vi "Configure Analog Output.vi"(6 "Enable Analog Output Reference (F: Disable)":bool, 7 "Analog Output Offset (0)":dbl, 8 "error in (no error)":errorcluster, 9 "Analog Output Gain (1)":dbl=1.0, 10 "Enable Analog Output (T: Enable)":bool=TRUE, 11 "VISA resource name":refnum<visa-resource-name>) -> (0 "error out":errorcluster, 3 "VISA resource name out":refnum<visa-resource-name>)   [LabVIEW 2011, in "Keithley 2182.lvlib"]
doc: "Configures the instrument's analog output. The analog output provides a scaled, non-inverting voltage output up to -1.2V and +1.2V. It is typically used to drive a chart recorder.\n\nThe Analog Output voltage is calculated as follows:\n\n<B>Analog Output = (Gain x Rdg/Rng) - Offset</B>\n\nwhere:\n<B>Gain</B> is the user entered gain factor.\n<B>Rdg</B> is the reading on the Model 2182.\n<B>Rng</B> is the measurement range.\n<B>Offset</B> is the user entered offset value."
uses:
  Keithley 2182.lvlib
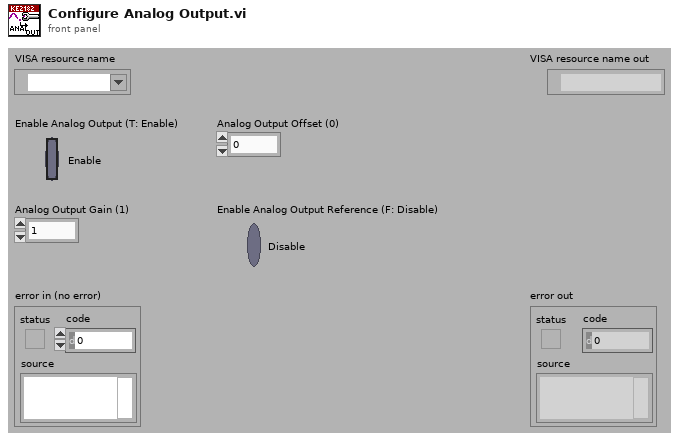
[diagram p1: front panel]
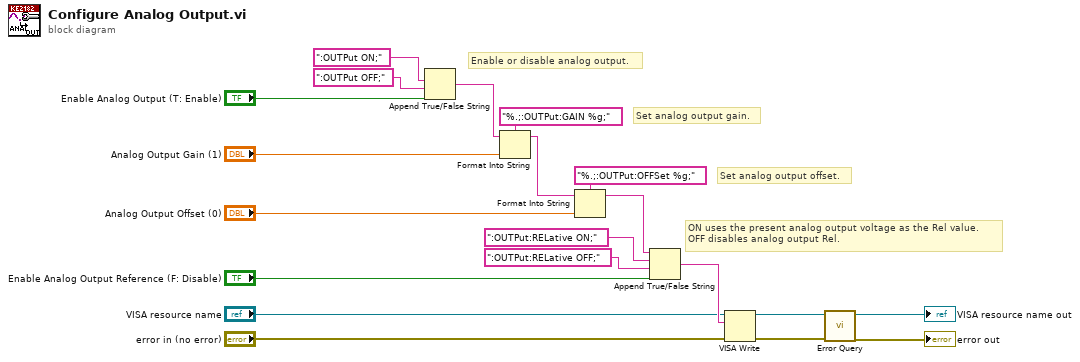
[diagram p0: block diagram]
diagram:
  # "ON uses the present analog output voltage as the Rel value.\nOFF disables analog output Rel."
  # "Set analog output offset."
  # "Set analog output gain."
  # "Enable or disable analog output."
  n1 = Append True/False String(1:"Enable Analog Output (T: Enable)", 2:":OUTPut OFF;", 3:":OUTPut ON;") -> (0:w17:string)  [unwired: 1 in]
  n2 = Format Into String(format string="%.;:OUTPut:GAIN %g;", initial string=w17, "Analog Output Gain (1)") -> (resulting string=w14:string)  [unwired: 1 in, 1 out]
  n3 = Format Into String(format string="%.;:OUTPut:OFFSet %g;", initial string=w14, "Analog Output Offset (0)") -> (resulting string=w11:string)  [unwired: 1 in, 1 out]
  n4 = Append True/False String(1:"Enable Analog Output Reference (F: Disable)", 2:":OUTPut:RELative OFF;", 3:":OUTPut:RELative ON;", 4:w11) -> (0:w7:string)
  n5 = VISA Write(VISA resource name="VISA resource name", write buffer=w7, error in (no error)="error in (no error)") -> (VISA resource name out=w4:refnum<visa-resource-name>, error out=w3:errorcluster)  [unwired: 1 out]
  n6 = call "Error Query.vi"("error in (no error)"=w3, "VISA resource name"=w4) -> ("error out"=→"error out":errorcluster, "VISA resource name out"=→"VISA resource name out":refnum<visa-resource-name>)  [unwired: 6 in, 2 out]
